vi "Word.vi"() -> ()   [LabVIEW 2015, in "Report.lvlib" / "Report - Word.lvlib"]
uses:
  Report - Word.lvlib
  <vilib>/Utility/NIReport.llb/image depth.ctl
  <vilib>/Utility/NIReport.llb/Append Report Text (str wrap).vi
  <vilib>/addons/_office/word.llb/Word Edit Cell ([str]).vi
  <vilib>/Utility/NIReport.llb/NI_report.lvclass
  <vilib>/Utility/NIReport.llb/Word/NI_Word.lvclass
  <vilib>/addons/_office/NI_ReportGenerationToolkit.lvlib
  <vilib>/Utility/NIReport.llb/NI_ReportGenerationCore.lvlib
panel:
  in  "Volt/Div B":u32(ring)=8 items=["10 mV", "20 mV", "50 mV", "100 mV", "200 mV", "500 mV", "1 V", "2 V", "5 V"]
  in  "Volt/Div A":u32(ring)=8 items=["10 mV", "20 mV", "50 mV", "100 mV", "200 mV", "500 mV", "1 V", "2 V", "5 V"]
  in  "TimeDiv":T1(ring)=enum."500us"
  out "Scope":waveform(dbl)[](graph)
  out "Pk-Pk(1)":dbl format="%#_g V"
  out "Freq(1)":dbl format="%#_g Hz"
  in  "Report":bool
  in  "§é dµi":string="1000"
  in  "Ng­êi ®o":string="Pham Nguyen Tong"
  in  "¸p suÊt":string="100"
  in  "§é Èm":string="70"
  in  "NhiÖt ®é":string="20"
  in  "Data":string[][](table)=[["100", "41.7", "38.5"], ["125", "41.7", "35.2"], ["160", "41.5", "37.5"], ["200", "42.3", "42.5"], ["250", "46.9", "46.8"], ["315", "51.9", "52.6"], ["400", "52.3", "46.7"], ["500  ", "46.5", "41.6"], ["630", "42.3", "35.9"], ["800", "41.1", "32.6"]]
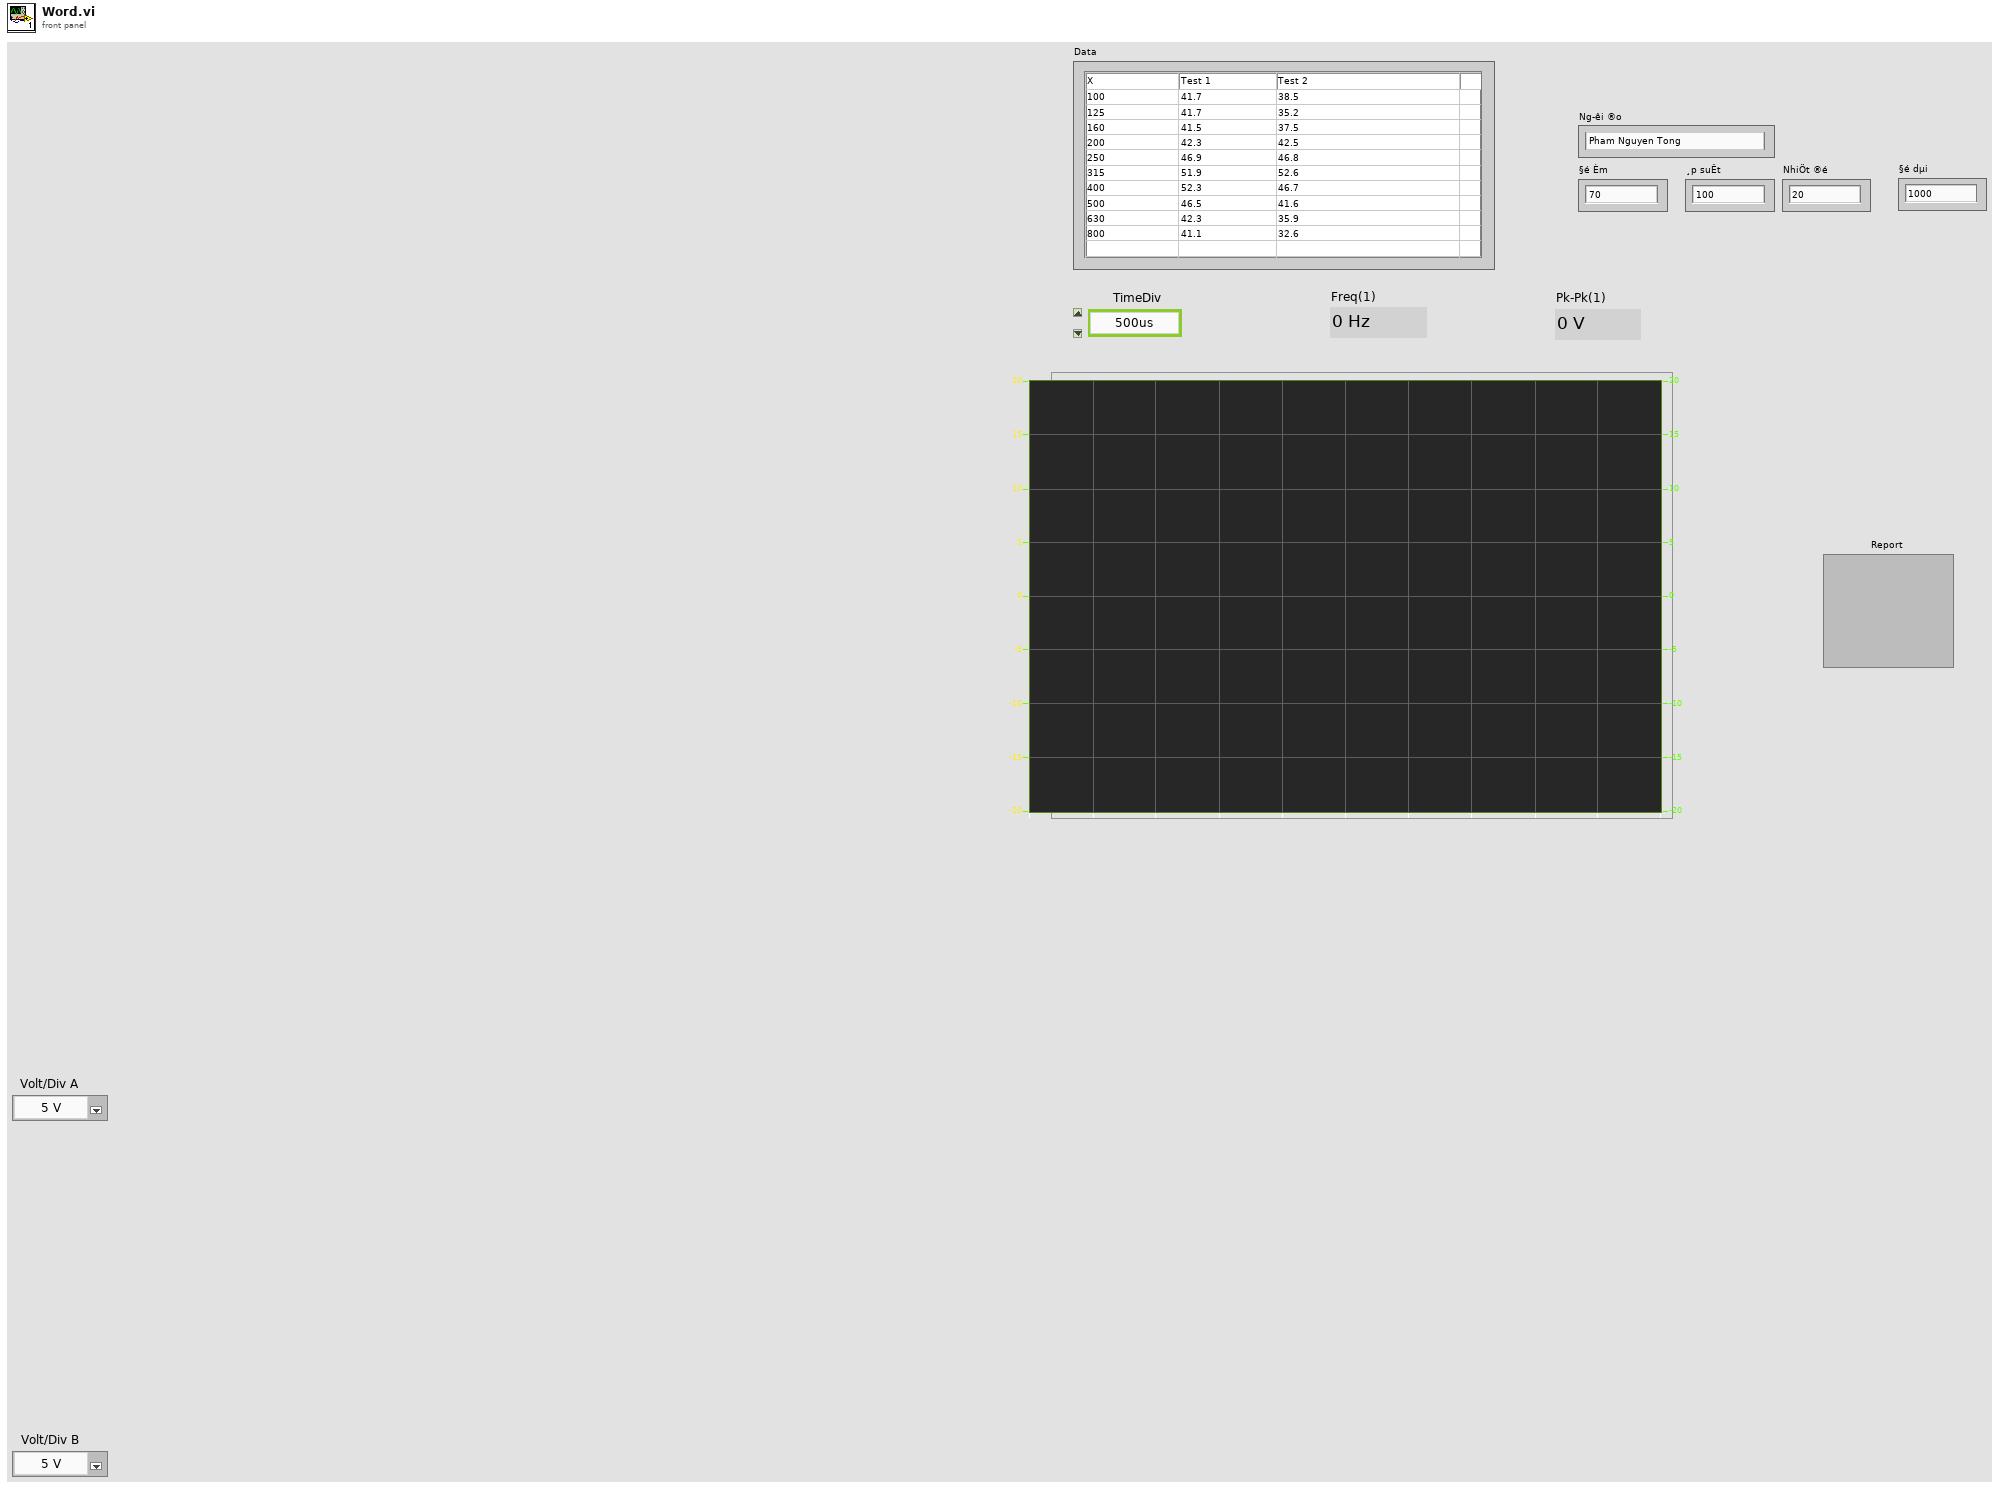
[diagram p1: front panel]
types:
  T1 = enum16{"100ms", "50ms", "20ms", "10ms", "5ms", "2ms", "1ms", "500us", "200us", "100us", "50us", "20us", "10us", "5us", "2us", "1us"}
  T2 = typedef "NI_ReportGenerationCore.lvlib/image depth.ctl" = u16
  T3 = cluster{"position (Excel)":cluster{"row":i32, "column":i32}, "name (Excel)":string, "bookmark (Word)":string}
  T4 = enum16{"Standard Report", "HTML", "Word", "Excel"}
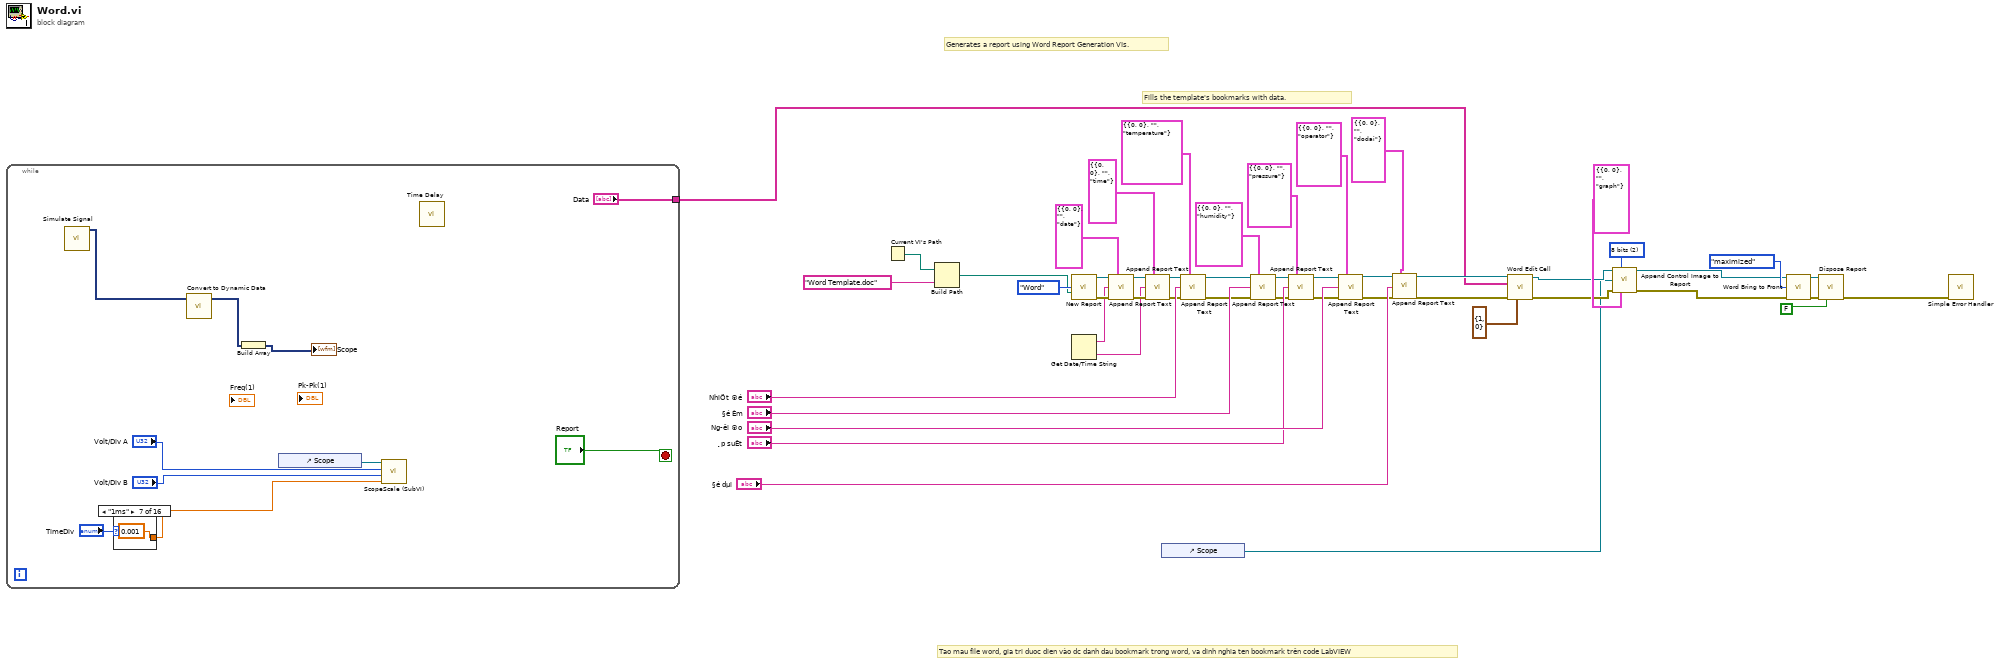
[diagram p0: block diagram]
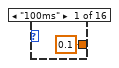
[diagram p2: hidden frame]
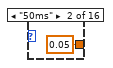
[diagram p3: hidden frame]
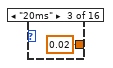
[diagram p4: hidden frame]
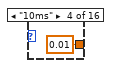
[diagram p5: hidden frame]
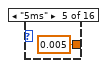
[diagram p6: hidden frame]
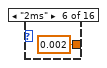
[diagram p7: hidden frame]
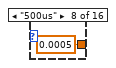
[diagram p8: hidden frame]
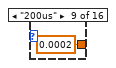
[diagram p9: hidden frame]
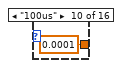
[diagram p10: hidden frame]
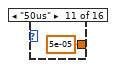
[diagram p11: hidden frame]
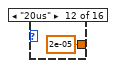
[diagram p12: hidden frame]
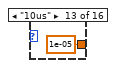
[diagram p13: hidden frame]
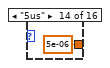
[diagram p14: hidden frame]
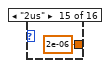
[diagram p15: hidden frame]
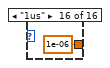
[diagram p16: hidden frame]
diagram:
  w10 = T2 2 items=["B&W", "4 bits", "8 bits", "24 bits"] ("image depth")
  # "Tao mau file word, gia tri duoc dien vào dc danh dau bookmark trong word, va dinh nghia ten bookmark trên code LabVIEW"
  # "Fills the template's bookmarks with data."
  # "Generates a report using Word Report Generation VIs."
  n1 = while {
    tunnel: ["Data"] -> w5
    stop <- "Report" stop-if-true
    n2 = call "Simulate Signal"() -> ("Square"=w50:dynamicdata)  [unwired: 14 in, 1 out]
    n3 = case shown="\"1ms\"" "TimeDiv" {
      tunnel: [0.1 0.05 0.02 0.01 0.005 0.002 0.001 0.0005 0.0002 0.0001 5e-05 2e-05 1e-05 5e-06 2e-06 1e-06] -> w55
      frame "100ms" {
      }
      frame "50ms" {
      }
      frame "20ms" {
      }
      frame "10ms" {
      }
      frame "5ms" {
      }
      frame "2ms" {
      }
      frame "1ms" {
      }
      frame "500us" {
      }
      frame "200us" {
      }
      frame "100us" {
      }
      frame "50us" {
      }
      frame "20us" {
      }
      frame "10us" {
      }
      frame "5us" {
      }
      frame "2us" {
      }
      frame "1us" {
      }
    }
    n4 = call "Convert to Dynamic Data"("Waveform"=w50) -> ("Dynamic Data Type"=w49:dynamicdata)  [unwired: 3 in]
    n5 = Build Array(w49) -> (→"Scope":dynamicdata[])
    n6 = control-ref of="Scope"() -> (w52:refnum<vi>)
    n7 = call "ScopeScale (SubVI).vi"("timeDiv"=w55, "VoltDivB"="Volt/Div B", "VoltDivA"="Volt/Div A", "Scope"=w52) -> ()  [unwired: 8 in]
    n8 = call "Time Delay"() -> ()  [unwired: 11 in, 1 out]
  }
  n9 = Current VI's Path() -> (path=w3:path)
  n10 = Build Path(base path=w3, name or relative path="Word Template.doc") -> (appended path=w2:path)
  n11 = call <vilib>:"New Report.vi"("report type"=T4."Word", "template (empty)"=w2) -> ("report out"=w35:refnum<class "NI_report.lvclass">, "error out"=w41:errorcluster)  [unwired: 12 in]
  n12 = Get Date/Time String() -> (date string=w17:string, time string=w18:string)  [unwired: 3 in]
  n13 = call-poly <vilib>:"Append Report Text.vi"("report in"=w35, "MS Office parameters"=T3 {"position (Excel)"={"row"=0, "column"=0}, "name (Excel)"="", "bookmark (Word)"="date"}, "text"=w17, "error in (no error)"=w41) -> ("report out"=w34:refnum<class "NI_report.lvclass">, "error out"=w40:errorcluster)  [unwired: 8 in, 2 out]
  n14 = call-poly <vilib>:"Append Report Text.vi"("report in"=w34, "MS Office parameters"=T3 {"position (Excel)"={"row"=0, "column"=0}, "name (Excel)"="", "bookmark (Word)"="time"}, "text"=w18, "error in (no error)"=w40) -> ("report out"=w33:refnum<class "NI_report.lvclass">, "error out"=w39:errorcluster)  [unwired: 8 in, 2 out]
  n15 = control-ref of="Scope"() -> (w4:refnum<vi>)
  n16 = call-poly <vilib>:"Append Report Text.vi"("report in"=w33, "MS Office parameters"=T3 {"position (Excel)"={"row"=0, "column"=0}, "name (Excel)"="", "bookmark (Word)"="temperature"}, "text"="NhiÖt ®é", "error in (no error)"=w39) -> ("report out"=w32:refnum<class "NI_report.lvclass">, "error out"=w38:errorcluster)  [unwired: 8 in, 2 out]
  n17 = call-poly <vilib>:"Append Report Text.vi"("report in"=w32, "MS Office parameters"=T3 {"position (Excel)"={"row"=0, "column"=0}, "name (Excel)"="", "bookmark (Word)"="humidity"}, "text"="§é Èm", "error in (no error)"=w38) -> ("report out"=w31:refnum<class "NI_report.lvclass">, "error out"=w37:errorcluster)  [unwired: 8 in, 2 out]
  n18 = call-poly <vilib>:"Append Report Text.vi"("report in"=w31, "MS Office parameters"=T3 {"position (Excel)"={"row"=0, "column"=0}, "name (Excel)"="", "bookmark (Word)"="pressure"}, "text"="¸p suÊt", "error in (no error)"=w37) -> ("report out"=w30:refnum<class "NI_report.lvclass">, "error out"=w36:errorcluster)  [unwired: 8 in, 2 out]
  n19 = call-poly <vilib>:"Append Report Text.vi"("report in"=w30, "MS Office parameters"=T3 {"position (Excel)"={"row"=0, "column"=0}, "name (Excel)"="", "bookmark (Word)"="operator"}, "text"="Ng­êi ®o", "error in (no error)"=w36) -> ("report out"=w16:refnum<class "NI_report.lvclass">, "error out"=w15:errorcluster)  [unwired: 8 in, 2 out]
  n20 = call-poly <vilib>:"Append Report Text.vi"("report in"=w16, "MS Office parameters"=T3 {"position (Excel)"={"row"=0, "column"=0}, "name (Excel)"="", "bookmark (Word)"="dodai"}, "text"="§é dµi", "error in (no error)"=w15) -> ("report out"=w14:refnum<class "NI_report.lvclass">, "error out"=w13:errorcluster)  [unwired: 8 in, 2 out]
  n21 = call-poly <vilib>:"Word Edit Cell.vi"("report in"=w14, "value"=w5, "error in (no error)"=w13, "start (0, 0)"=cluster{"row":i32, "column":i32} {"row"=1, "column"=0}) -> ("report out"=w9:refnum<class "NI_report.lvclass">, "error out"=w8:errorcluster)  [unwired: 10 in]
  n22 = call-dynamic "Append Control Image to Report.vi"("report in"=w9, "image depth"=w10, "ctrl reference"=w4, "error in (no error)"=w8, "MS Office parameters"=T3 {"position (Excel)"={"row"=0, "column"=0}, "name (Excel)"="", "bookmark (Word)"="graph"}) -> ("report out"=w7:refnum<class "NI_report.lvclass">, "error out"=w6:errorcluster)  [unwired: 7 in, 2 out]
  n23 = call <vilib>:"Word Bring to Front.vi"("report in"=w7, "window state (maximized)"=enum16{"maximized", "minimized", "normal"}."maximized", "error in (no error)"=w6) -> ("report out"=w21:refnum<class "NI_report.lvclass">, "error out"=w22:errorcluster)  [unwired: 11 in]
  n24 = call-dynamic "Dispose Report.vi"("report in"=w21, "error in (no error)"=w22, "close report? (T)"=FALSE ("Close Report? (T)")) -> ("error out"=w45:errorcluster)  [unwired: 12 in]
  n25 = call <vilib>:"Simple Error Handler.vi"("error in (no error)"=w45) -> ()  [unwired: 4 in, 5 out]
